vi "to q10.vi"(2 "Food Item In":T1 {"Q" format="%.1f"; "FEP"."PSY"."+2" format="%#.2f"; "FEP"."PSY"."+1" format="%#.2f"; "FEP"."WIL"."+2" format="%#.2f"; "FEP"."WIL"."+1" format="%#.2f"; "FEP"."DEX"."+2" format="%#.2f"; "FEP"."DEX"."+1" format="%#.2f"; "FEP"."CHA"."+2" format="%#.2f"; "FEP"."CHA"."+1" format="%#.2f"; "FEP"."PRC"."+2" format="%#.2f"; "FEP"."PRC"."+1" format="%#.2f"; "FEP"."CON"."+2" format="%#.2f"; "FEP"."CON"."+1" format="%#.2f"; "FEP"."INT"."+2" format="%#.2f"; "FEP"."INT"."+1" format="%#.2f"; "FEP"."AGI"."+2" format="%#.2f"; "FEP"."AGI"."+1" format="%#.2f"; "FEP"."STR"."+2" format="%#.2f"; "FEP"."STR"."+1" format="%#.2f"; "Energy" format="%.0f%"; "Hunger" format="%#.2f%"}) -> (6 "Food Item Out":T1 {"Q" format="%.1f"; "FEP"."PSY"."+2" format="%#.2f"; "FEP"."PSY"."+1" format="%#.2f"; "FEP"."WIL"."+2" format="%#.2f"; "FEP"."WIL"."+1" format="%#.2f"; "FEP"."DEX"."+2" format="%#.2f"; "FEP"."DEX"."+1" format="%#.2f"; "FEP"."CHA"."+2" format="%#.2f"; "FEP"."CHA"."+1" format="%#.2f"; "FEP"."PRC"."+2" format="%#.2f"; "FEP"."PRC"."+1" format="%#.2f"; "FEP"."CON"."+2" format="%#.2f"; "FEP"."CON"."+1" format="%#.2f"; "FEP"."INT"."+2" format="%#.2f"; "FEP"."INT"."+1" format="%#.2f"; "FEP"."AGI"."+2" format="%#.2f"; "FEP"."AGI"."+1" format="%#.2f"; "FEP"."STR"."+2" format="%#.2f"; "FEP"."STR"."+1" format="%#.2f"; "Energy" format="%.0f%"; "Hunger" format="%#.2f%"})   [LabVIEW 2018]
uses:
  FoodItem.ctl
  FEP.ctl
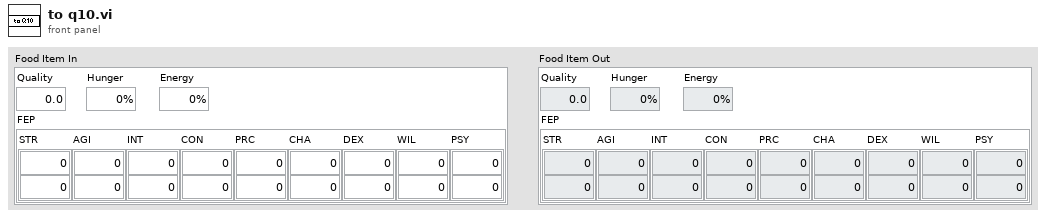
[diagram p1: front panel]
types:
  T1 = typedef "FoodItem.ctl" = cluster{"Q":dbl, "Hunger":dbl, "Energy":i32, "FEP":T2}
  T2 = typedef "FEP.ctl" = cluster{"STR":cluster{"+1":dbl, "+2":dbl}, "AGI":cluster{"+1":dbl, "+2":dbl}, "INT":cluster{"+1":dbl, "+2":dbl}, "CON":cluster{"+1":dbl, "+2":dbl}, "PRC":cluster{"+1":dbl, "+2":dbl}, "CHA":cluster{"+1":dbl, "+2":dbl}, "DEX":cluster{"+1":dbl, "+2":dbl}, "WIL":cluster{"+1":dbl, "+2":dbl}, "PSY":cluster{"+1":dbl, "+2":dbl}}
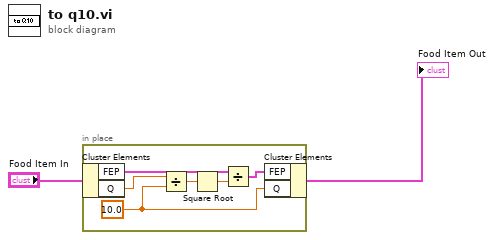
[diagram p0: block diagram]
diagram:
  n1 = in-place {
    w3 = 10.0 ("y")
    n2 = in-place-cluster #1("Food Item In") -> ("FEP"=w7:T2, "Q"=w6:dbl)
    n3 = Divide(x=w6, y=w3) -> (x/y=w8:dbl)
    n4 = Square Root(x=w8) -> (sqrt(x)=w5:dbl)
    n5 = Divide(x=w7, y=w5) -> (x/y=w4:T2)
    n6 = in-place-cluster #1("FEP"=w4, "Q"=w3) -> (→"Food Item Out":T1)
  }
